vi "Enable Disable Controls.vi"(8 "error in (no error)":errorcluster, 10 "Disabled":T1(ring), 11 "Control Refnum":refnum<vi>[](array[refnum])) -> (0 "Error Out":errorcluster)   [LabVIEW 2024]
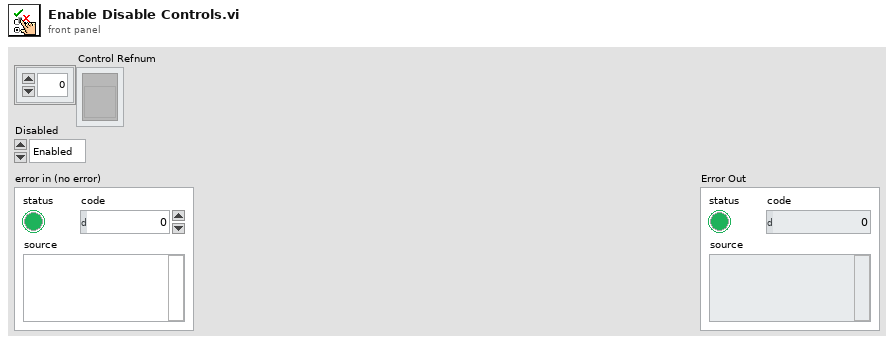
[diagram p1: front panel]
types:
  T1 = enum8{"Enabled", "Disabled", "Disabled and Grayed Out"}
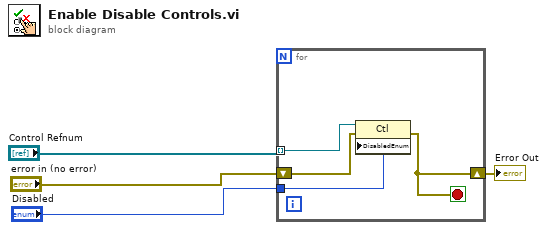
[diagram p0: block diagram]
diagram:
  n1 = for {
    tunnel: "Control Refnum" -> [w8] mode=indexing
    shift-right: [w6] -> w2
    shift-left: "error in (no error)" -> [w7]
    tunnel: "Disabled" -> [w5]
    stop <- w6 stop-if-true
    n2 = property class="Ctl"(reference=w8, error in=w7, "DisabledEnum"=w5) -> (error out=w6:errorcluster)  [unwired: 1 out]
  }
  "Error Out" <- w2
